vi "Init Node Info.vi"(6 "App Version":string, 8 "error in (no error)":errorcluster, 11 "DiscoveryService in":refnum<class "DiscoveryService.lvclass">) -> (0 "error out":errorcluster, 3 "DiscoveryService out":refnum<class "DiscoveryService.lvclass">)   [LabVIEW 2020, in "Vecto.lvlib" / "DiscoveryService.lvclass"]
uses:
  DiscoveryService.lvclass
  DiscoveryService.lvclass/DiscoveryService.ctl
  lv-volatus/messages/ServiceType/Enumeration.ctl
  lv-volatus/messages/ServiceType/ServiceType.lvlib
  lv-volatus/messages/Service/Data.ctl
  lv-volatus/messages/Service/Service.lvlib
  lv-volatus/messages/Discovery/Data.ctl
  lv-volatus/messages/Discovery/Discovery.lvlib
  Node Config/Node Config.lvclass
  lv-volatus/messages/Discovery/Class/Msg.lvclass
  Vecto.lvlib
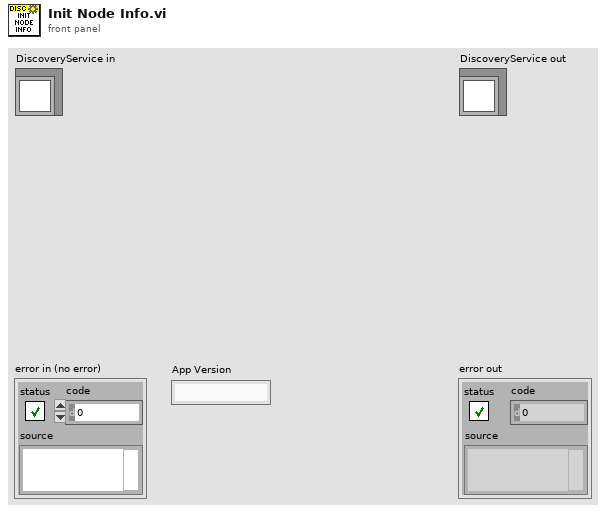
[diagram p1: front panel]
types:
  T1 = typedef "Discovery.lvlib/Data.ctl" = cluster{"node_id":u32, "name":string, "ip":u32, "status":string, "services":T2[], "capabilities":string[], "system":string, "cluster":string, "app_version":string, "cfg_version":string}
  T2 = typedef "Service.lvlib/Data.ctl" = cluster{"type":T3, "port":i32}
  T3 = typedef "ServiceType.lvlib/Enumeration.ctl" = enum16{"SERVICETYPE_UNKNOWN", "SERVICETYPE_TCPSERVER", "SERVICETYPE_HTTPSERVER"}
  T4 = typedef "VectoConfig.lvlib/Discovery Info.ctl" = cluster{"Address":string, "Port":u16, "Interval S":dbl, "Bind Address":string}
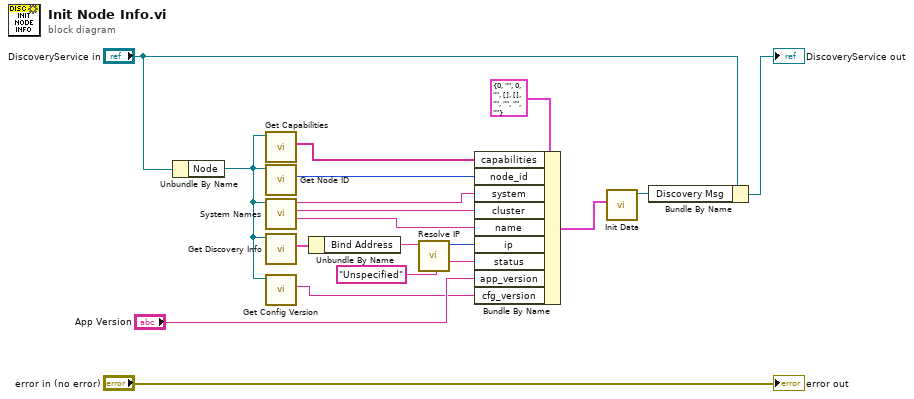
[diagram p0: block diagram]
diagram:
  n1 = Unbundle By Name("DiscoveryService in") -> ("Node"=w4:refnum<class "Node Config.lvclass">)
  n2 = call "Get Capabilities.vi"("Node Config in"=w4) -> ("Capabilities"=w5:string[])  [unwired: 8 in, 2 out]
  n3 = call "Get Node ID.vi"("Node in"=w4) -> ("Node ID"=w17:u32)  [unwired: 8 in, 2 out]
  n4 = call "System Names.vi"("Node Config in"=w4) -> ("Name"=w9:string, "Cluster"=w8:string, "System"=w7:string)  [unwired: 8 in]
  n5 = call "Get Discovery Info.vi"("Node in"=w4) -> ("Discovery Info"=w10:T4)  [unwired: 8 in, 2 out]
  n6 = call "Get Config Version.vi"("Node Config in"=w4) -> ("Config Version"=w3:string)  [unwired: 8 in, 2 out]
  n7 = Unbundle By Name(w10) -> ("Bind Address"=w2:string)
  n8 = call "Resolve IP.vi"("Address In"=w2) -> ("U32 Address"=w1:u32)  [unwired: 8 in, 2 out]
  n9 = Bundle By Name(cluster=T1 {"node_id"=0, "name"="", "ip"=0, "status"="", "services"=[], "capabilities"=[], "system"="", "cluster"="", "app_version"="", "cfg_version"=""} ("Discovery"), "capabilities"=w5, "node_id"=w17, "system"=w7, "cluster"=w8, "name"=w9, "ip"=w1, "status"="Unspecified", "app_version"="App Version", "cfg_version"=w3) -> (w15:T1)
  n10 = call "Init Data.vi"("Data"=w15) -> ("Msg out"=w13:refnum<class "Msg.lvclass">)  [unwired: 10 in]
  n11 = Bundle By Name(cluster="DiscoveryService in", "Discovery Msg"=w13) -> (→"DiscoveryService out":refnum<class "DiscoveryService.lvclass">)
  "error out" <- "error in (no error)"
